vi "balance.vi"() -> ()   [LabVIEW 2013]
uses:
  <vilib>/Analysis/NI_AALBase.lvlib
  <vilib>/Instr/_visa.llb/VISA Configure Serial Port (Instr).vi
  <vilib>/Analysis/3filter.llb/Savitzky-Golay Filter (DBL).vi
  <vilib>/Analysis/3filter.llb/FIR Filter (DBL).vi
  <vilib>/Analysis/3filter.llb/Zero Phase Filter (DBL).vi
  <vilib>/measure/maspectr.llb/FFT Spectrum (Mag-Phase).vi
  <vilib>/measure/NI_MAPro.lvlib
  <vilib>/robotics/Controls/2D Rangefinder/NI_Robotics_2D Rangefinder.xctl
panel:
  in  "PWM":u16(knob) scale=1100.0..1900.0
  in  "Направление\nвращения":dbl=-1.0
  in  "Усиление расчетной фазы":dbl(slide)=0.02993150684931507 scale=0.005..0.04
  in  "Правка фазы":dbl(slide)=105.29268292682927 scale=0.0..360.0
  in  "0 акселер.":dbl
  in  "Выбор т.":bool
  out "max а":i32
  out "по обор.":i32
  out "Рабочий диапозон":waveform(dbl)(graph)
  in  "использование\n ф. сигнала":bool
  out "Расчетные \nзначения":cluster{"angle":dbl[], "distance":dbl[][]}(xcontrol)
  out "Расчетный спектр на основе БПФ":cluster{"f0":dbl, "df":dbl, "magnitude":dbl[]}(graph)
  in  "Сглаживание":T1(ring)
  in  "Правка фазы":dbl(slide) scale=0.0..360.0
  in  "Усиление уровня мигнала":dbl(slide)=0.014857142857142857 scale=0.005..0.02
  out "N об.":i32
  out "Об/мин":dbl(knob) scale=0.0..6000.0
  out "Ф. сигнал\n в полярных \nкоординатах":cluster{"angle":dbl[], "distance":dbl[][]}(xcontrol)
  in  "Вывод\nновых\nданных":bool
  in  "side points":i32(slide)=20 scale=0.0..40.0
  in  "polynomial order":i32(slide)=2 scale=0.0..20.0
  out "Сигнал со стенда":cluster{i32[], dbl[]}[](graph)
  in  "Выбор фильтра":u16(ring) items=["Savetzky-Golay", "Median", "FIR", "Zero Fhase"]
  in  "второй":i32=2
  in  "Установка скорости":u32=115200
  in  "Выбор порта":refnum<visa-resource-name>="COM13"
  out "данные из порта":string
  out "Отфильтрованный сигнал":cluster{i32[], "Filtered X":dbl[]}[](graph)
  in  "stop":bool
  # "0"
  # "180"
  # "F12"
  # "первый"
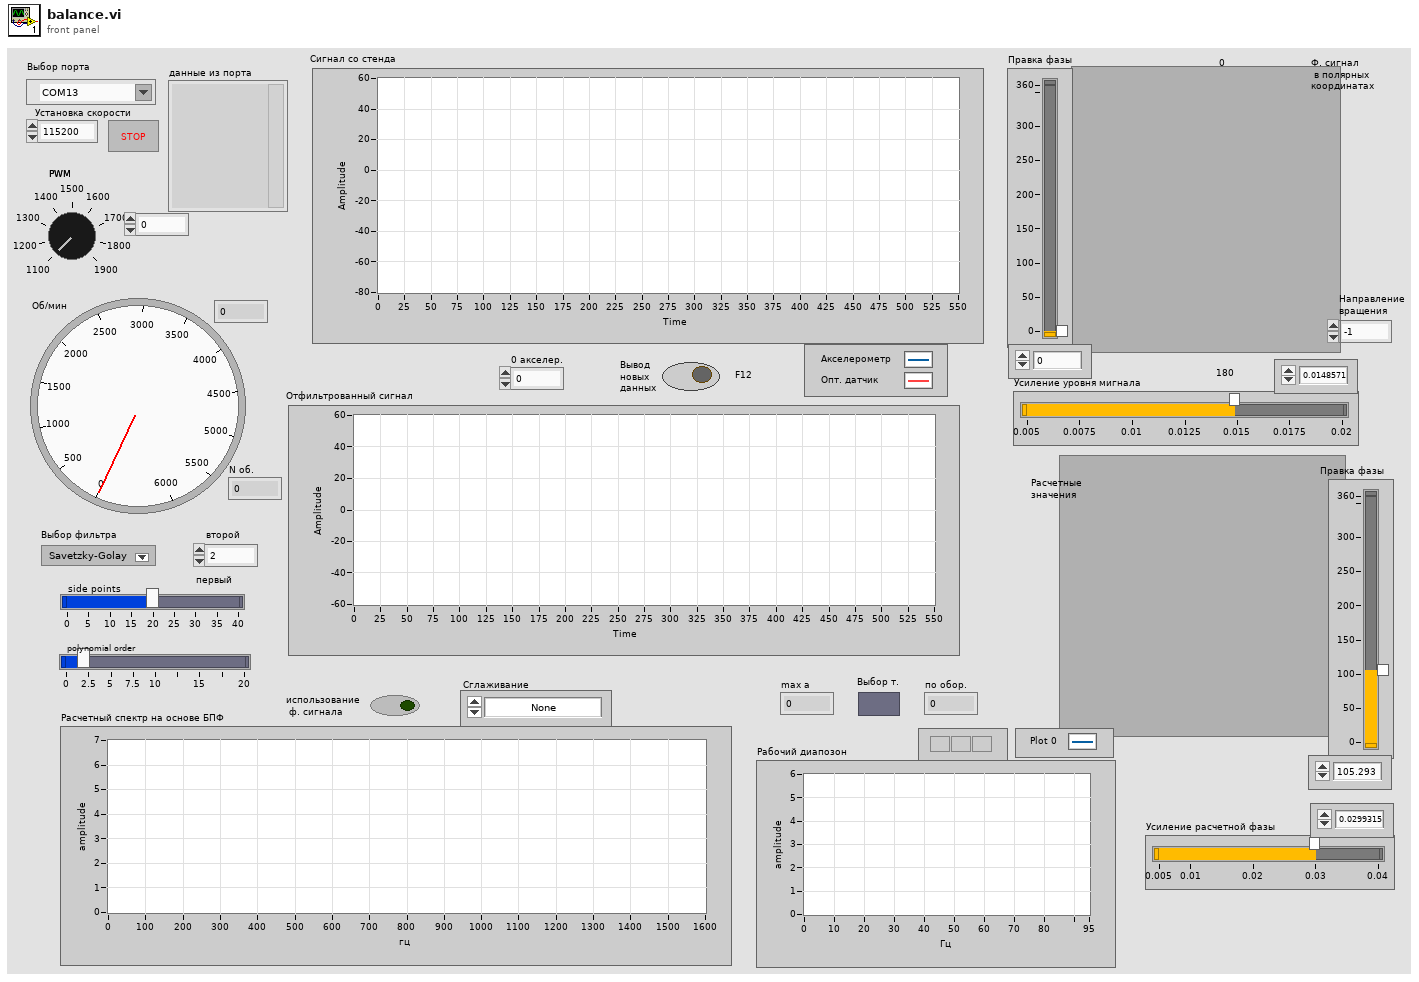
[diagram p1: front panel]
types:
  T1 = enum16{"None ", "Hanning", "Hamming", "Blackman-Harris", "Exact Blackman", "Blackman", "Flat Top", "4 Term B-Harris ", "7 Term B-Harris", "Low Sidelobe"}
  T2 = cluster{"dB On (F)":bool, "unwrap phase (F)":bool, "convert to degree (F)":bool}
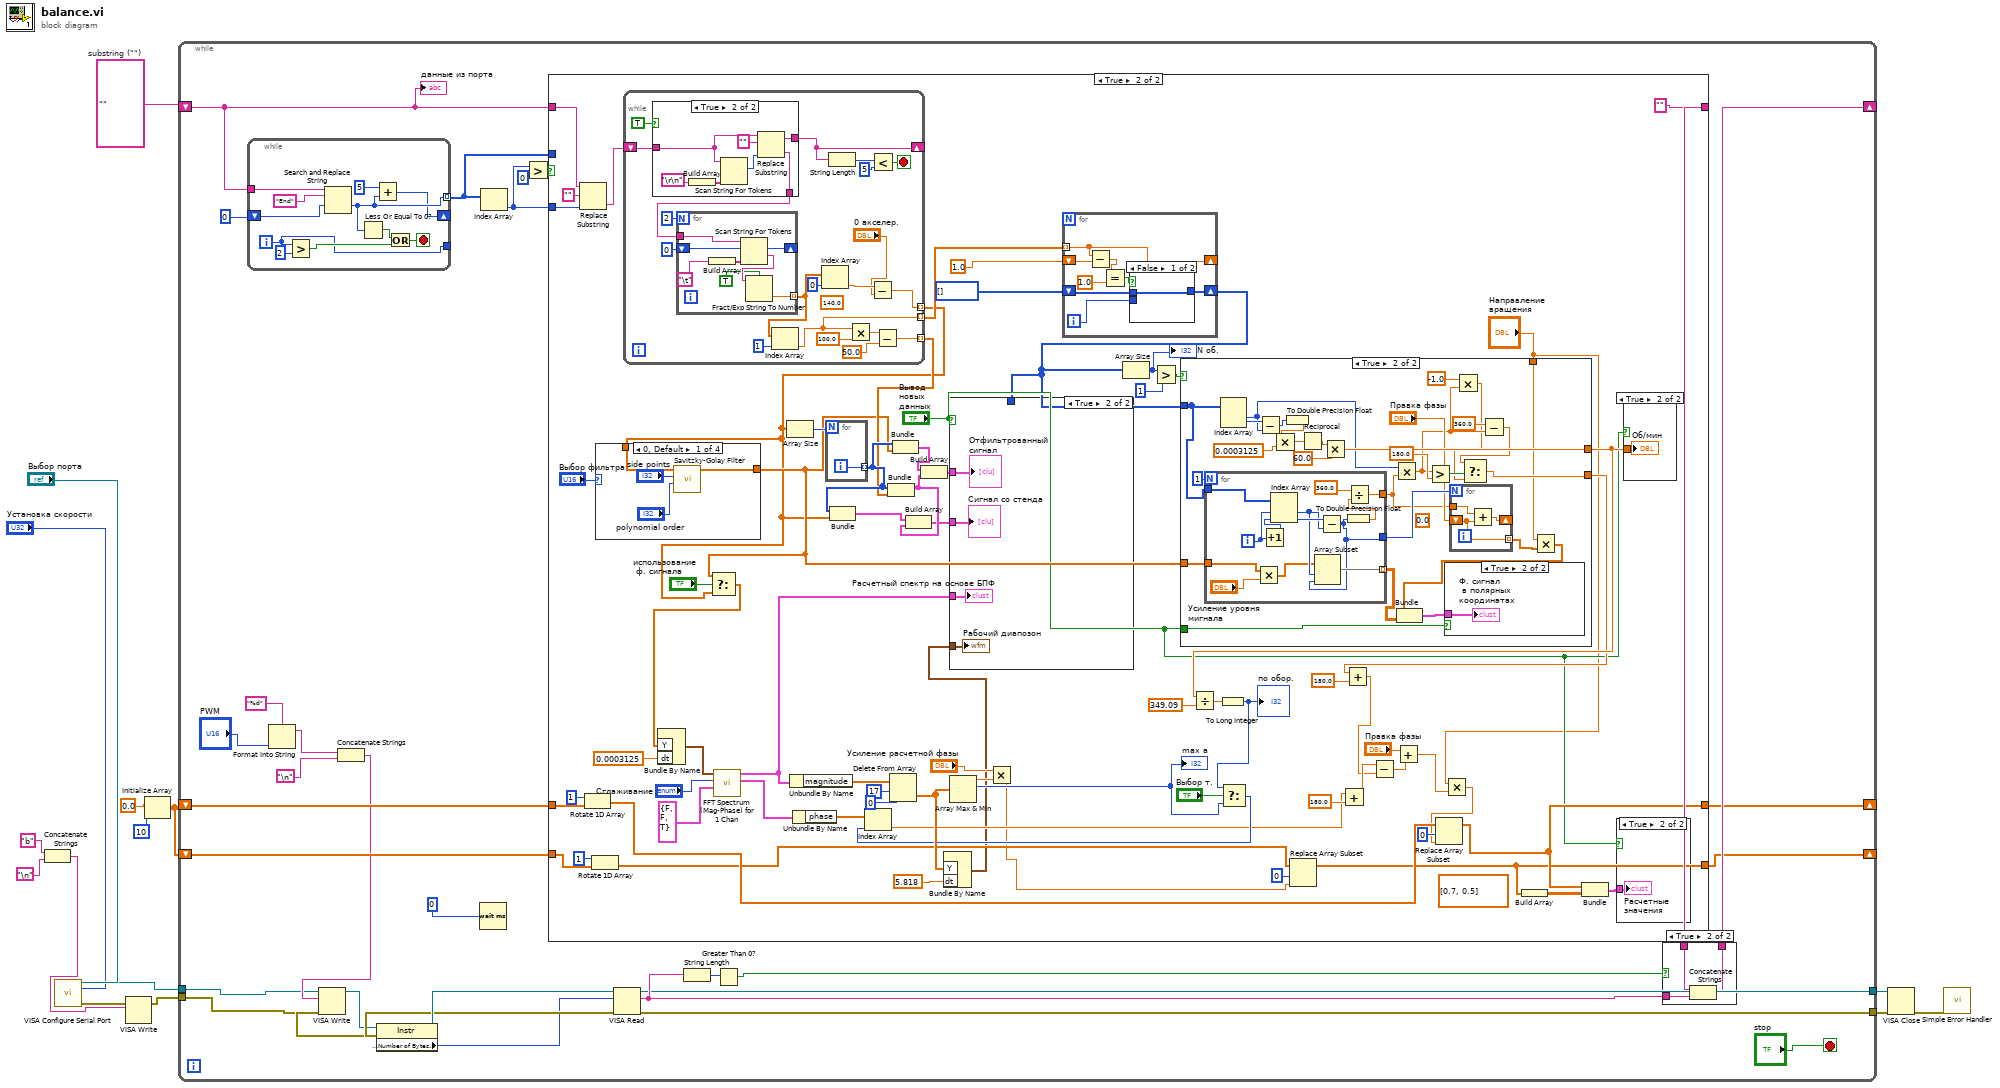
[diagram p0: block diagram]
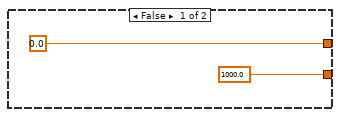
[diagram p6: hidden frame]
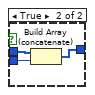
[diagram p8: hidden frame]
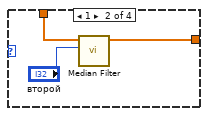
[diagram p10: hidden frame]
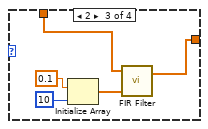
[diagram p11: hidden frame]
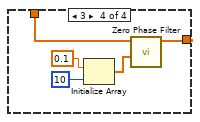
[diagram p12: hidden frame]
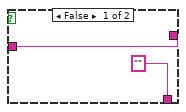
[diagram p13: hidden frame]
diagram:
  w12 = ""  # substring ("")
  n1 = Concatenate Strings("b", "\n") -> (w1:string)
  n2 = call-poly "VISA Configure Serial Port"("VISA resource name"="Выбор порта", "baud rate (9600)"="Установка скорости") -> ("VISA resource name out"=w11:refnum<visa-resource-name>, "error out"=w10:errorcluster)  [unwired: 7 in, 5 out]
  n3 = VISA Write(write buffer=w1) -> ()  [unwired: 2 in, 3 out]
  n4 = Initialize Array(0.0, 10 ("dimension size")) -> (w4:dbl[])
  n5 = while {
    shift-right: [w33] -> _
    shift-left: w12 -> [w30]
    tunnel: w11 -> [w15]
    tunnel: w10 -> [w16]
    tunnel: [w32] -> w8
    tunnel: [w31] -> w7
    shift-right: [w26] -> _
    shift-left: w4 -> [w27]
    shift-right: [w24] -> _
    shift-left: w4 -> [w25]
    stop <- "stop" stop-if-true
    n6 = while {
      tunnel: w30 -> [w256]
      shift-right: [w252] -> _
      shift-left: 0 -> [w251]
      tunnel: [w254] -> w29 mode=indexing
      tunnel: [w246] -> _
      i -> [w246]
      stop <- w247 stop-if-true
      n7 = Greater?(x=w246, y=2) -> (0:w248:bool)
      n8 = Search and Replace String(input string=w256, search string="End", offset=w251) -> (offset past replacement=w254:i32)  [unwired: 5 in, 3 out]
      n9 = Less Or Equal To 0?(x=w254) -> (x <= 0?=w250:bool)
      n10 = Add(x=5, y=w254) -> (x+y=w252:i32)
      n11 = Or(x=w250, y=w248) -> (x .or. y?=w247:bool)
    }
    n12 = Format Into String(format string="%d", "PWM") -> (resulting string=w19:string)  [unwired: 2 in, 1 out]
    n13 = Concatenate Strings(w19, "\n") -> (w17:string)
    n14 = VISA Write(VISA resource name=w15, write buffer=w17, error in (no error)=w16) -> (VISA resource name out=w22:refnum<visa-resource-name>, error out=w23:errorcluster)  [unwired: 1 out]
    n15 = property class="Instr"(reference=w22, error in=w23) -> (reference out=w40:refnum<visa-resource-name>, error out=w39:errorcluster, "Serial Settings:Number of Bytes at Serial Port"=w38:u32)
    n16 = Wait (ms)(milliseconds to wait=u32 0) -> ()  [unwired: 1 out]
    n17 = Index Array(array=w29) -> (element=w28:i32)  [unwired: 1 in]
    n18 = Greater?(x=w28, y=0) -> (0:w41:bool)
    n19 = case shown="True" w41 {
      tunnel: w29 -> [_ _]
      tunnel: [w52 ""] -> w34
      tunnel: w30 -> [w52 w122]
      tunnel: w28 -> [_ w120]
      tunnel: w27 -> [w51 w73]
      tunnel: [w51 w69] -> w26
      tunnel: w25 -> [w50 w67]
      tunnel: [w50 w61] -> w24
      frame False {
      }
      frame True {
        (unwired) dbl[][] [[0.7, 0.5]]
        n20 = Replace Substring(2:w120, 4:"" ("substring (\"\")"), 5:w122) -> (0:w119:string)  [unwired: 1 in, 1 out]
        n21 = Rotate 1D Array(1:w73, 2:1 ("n")) -> (0:w71:dbl[])
        n22 = Rotate 1D Array(1:w67, 2:1 ("n")) -> (0:w65:dbl[])
        n23 = while {
          shift-right: [w223] -> _
          shift-left: w119 -> [w226]
          tunnel: [w211] -> w95 mode=indexing
          tunnel: [w216] -> w103 mode=indexing
          tunnel: [w213] -> w109 mode=indexing
          stop <- w220 stop-if-true
          (unwired) 140.0
          n24 = case shown="True" TRUE {
            tunnel: [w230 w234] -> w223
            tunnel: w226 -> [w230 w233]
            tunnel: ["" w231] -> w225
            frame False {
            }
            frame True {
              n25 = Build Array("\r\n") -> (w236:string[])
              n26 = Scan String For Tokens(6:w236, 9:w233) -> (2:w232:i32)  [unwired: 4 in, 3 out]
              n27 = Replace Substring(2:w232, 4:"" ("substring (\"\")"), 5:w233) -> (0:w231:string, 1:w234:string)  [unwired: 1 in]
            }
          }
          n28 = for {
            N: 2 -> [_]
            tunnel: w225 -> [w244]
            shift-right: [w243] -> _
            shift-left: 0 -> [w242]
            tunnel: [w240] -> w214 mode=indexing
            n29 = Build Array("\t") -> (w245:string[])
            n30 = Scan String For Tokens(6:w245, 8:w242, 9:w244) -> (1:w241:string, 2:w243:i32)  [unwired: 3 in, 2 out]
            n31 = Fract/Exp String To Number(use system decimal point (T)=TRUE, string=w241) -> (number=w240:dbl)  [unwired: 2 in, 1 out]
          }
          n32 = Index Array(array=w214, index=1) -> (element=w213:dbl)
          n33 = Index Array(array=w214, index=0) -> (element=w212:dbl)
          n34 = String Length(string=w223) -> (length=w222:i32)
          n35 = Multiply(x=w213, y=100.0) -> (x*y=w218:dbl)
          n36 = Subtract(x=w212, y="0 акселер.") -> (x-y=w211:dbl)
          n37 = Less?(x=w222, y=5) -> (x < y?=w220:bool)
          n38 = Subtract(x=w218, y=50.0) -> (x-y=w216:dbl)
        }
        n39 = case shown="0, Default" "Выбор фильтра" {
          tunnel: w95 -> [w194 w197 w199 w205]
          tunnel: [w193 w195 w198 w204] -> w96
          frame 0, Default {
            n40 = call-poly <vilib>:"Savitzky-Golay Filter.vi"("polynomial order"="polynomial order", "side points"="side points", "X"=w194) -> ("Filtered X"=w193:dbl[])  [unwired: 7 in, 1 out]
          }
          frame 1 {
            n41 = call <vilib>:"Median Filter.vi"("left rank"="второй", "X"=w197) -> ("Filtered X"=w195:dbl[])  [unwired: 8 in, 1 out]
          }
          frame 2 {
            n42 = Initialize Array(0.1 ("element"), 10 ("dimension size")) -> (w200:dbl[])
            n43 = call-poly <vilib>:"FIR Filter.vi"("FIR Coefficients"=w200, "X"=w199) -> ("Filtered X"=w198:dbl[])  [unwired: 2 in, 1 out]
          }
          frame 3 {
            n44 = Initialize Array(0.1 ("element"), 10 ("dimension size")) -> (w206:dbl[])
            n45 = call-poly <vilib>:"Zero Phase Filter.vi"("Forward Coefficients"=w206, "X"=w205) -> ("Filtered X"=w204:dbl[])  [unwired: 8 in, 1 out]
          }
        }
        n46 = Select(t=w96, s="использование\n ф. сигнала", f=w95) -> (s? t:f=w94:dbl[])
        n47 = Bundle By Name("Y"=w94, "dt"=0.0003125) -> (w98:waveform(dbl))  [unwired: 1 in]
        n48 = call-poly <vilib>:"FFT Spectrum (Mag-Phase) for 1 Chan.vi"("view"=T2 {"dB On (F)"=FALSE, "unwrap phase (F)"=FALSE, "convert to degree (F)"=TRUE}, "window"="Сглаживание", "time signal"=w98) -> ("phase"=w83:cluster{"f0":dbl, "df":dbl, "phase":dbl[]}, "magnitude"=w59:cluster{"f0":dbl, "df":dbl, "magnitude":dbl[]})  [unwired: 4 in, 3 out]
        n49 = Array Size(array=w95) -> (size(s)=w107:i32)
        n50 = Unbundle By Name(w59) -> ("magnitude"=w93:dbl[])
        n51 = Unbundle By Name(w83) -> ("phase"=w97:dbl[])
        n52 = for {
          N: w107 -> [_]
          tunnel: [w208] -> w117 mode=indexing
          i -> [w208]
        }
        n53 = Bundle(w117, w95) -> (w118:cluster{i32[], dbl[]})  [unwired: 1 in]
        n54 = Bundle(w117, w103) -> (w116:cluster{i32[], dbl[]})  [unwired: 1 in]
        n55 = Delete From Array(array=w93, length=17, index=0) -> (deleted portion=w88:dbl[])  [unwired: 1 out]
        n56 = Bundle(w117, "Filtered X"=w96) -> (w124:cluster{i32[], "Filtered X":dbl[]})  [unwired: 1 in]
        n57 = Build Array(w118, w116) -> (w115:cluster{i32[], dbl[]}[])
        n58 = Build Array(w124, w116) -> (w106:cluster{i32[], "Filtered X":dbl[]}[])
        n59 = Bundle By Name("Y"=w88, "dt"=5.818) -> (w57:waveform(dbl))  [unwired: 1 in]
        n60 = Array Max & Min(array=w88) -> (max value=w64:dbl, max index (indices)=w85:i32)  [unwired: 2 out]
        "max а" <- w85
        n61 = Multiply(x="Усиление расчетной фазы", y=w64) -> (x*y=w62:dbl)
        n62 = for {
          tunnel: w109 -> [w181] mode=indexing
          shift-right: [w181] -> _
          shift-left: 1.0 -> [w182]
          shift-right: [w175] -> w56
          shift-left: i32[] [] -> [w176]
          i -> [w177]
          n63 = Subtract(x=w181, y=w182) -> (x-y=w180:dbl)
          n64 = Equal?(x=w180, y=1.0) -> (x = y?=w178:bool)
          n65 = case shown="False" w178 {
            tunnel: w177 -> [_ w186]
            tunnel: w176 -> [w183 w185]
            tunnel: [w183 w184] -> w175
            frame False {
            }
            frame True {
              n66 = Build Array (concatenate)(w185, w186) -> (w184:i32[])
            }
          }
        }
        n67 = case shown="True" "Вывод\nновых\nданных" {
          tunnel: w106 -> [_ w190]
          tunnel: w115 -> [_ w189]
          tunnel: w59 -> [_ w188]
          tunnel: w57 -> [_ w187]
          tunnel: w56 -> [_ _]
          frame False {
          }
          frame True {
            "Отфильтрованный сигнал" <- w190
            "Сигнал со стенда" <- w189
            "Расчетный спектр на основе БПФ" <- w188
            "Рабочий диапозон" <- w187
          }
        }
        n68 = Array Size(array=w56) -> (size(s)=w108:i32)
        "N об." <- w108
        n69 = Greater?(x=w108, y=1) -> (0:w110:bool)
        n70 = case shown="True" w110 {
          tunnel: w56 -> [_ w151]
          tunnel: [0.0 w152] -> w102
          tunnel: w96 -> [_ w142]
          tunnel: "Вывод\nновых\nданных" -> [_ w144]
          tunnel: [1000.0 w132] -> w82
          tunnel: "Направление\nвращения" -> [_ w129]
          frame False {
          }
          frame True {
            (unwired) 0.0
            n71 = for {
              N: 1 -> [_]
              tunnel: w151 -> [w172]
              tunnel: w142 -> [w164]
              tunnel: [w167] -> w146 mode=indexing
              tunnel: [w166] -> w145
              tunnel: [w165] -> w141
              i -> [w173]
              n72 = Multiply(x=w164, y="Усиление уровня мигнала") -> (x*y=w163:dbl[])
              n73 = Increment(x=w173) -> (x+1=w174:i32)
              n74 = Index Array(array=w172, index #1=w173, index #2=w174) -> (element #1=w168:i32, element #2=w169:i32)
              n75 = Subtract(x=w169, y=w168) -> (x-y=w166:i32)
              n76 = Array Subset(array=w163, index=w168, length=w166) -> (w167:dbl[])
              n77 = To Double Precision Float(number=w166) -> (double precision float=w170:dbl)
              n78 = Divide(x=360.0, y=w170) -> (x/y=w165:dbl)
            }
            n79 = Index Array(array=w151) -> (element #1=w140:i32, element #2=w157:i32)  [unwired: 2 in]
            n80 = Subtract(x=w157, y=w140) -> (x-y=w150:i32)
            n81 = To Double Precision Float(number=w150) -> (double precision float=w149:dbl)
            n82 = Multiply(x=w149, y=0.0003125 ("dt")) -> (x*y=w155:dbl)
            n83 = Reciprocal(x=w155) -> (1/x=w154:dbl)
            n84 = Multiply(x=w154, y=60.0) -> (x*y=w152:dbl)
            n85 = Multiply(x=w140, y=w141) -> (x*y=w135:dbl)
            n86 = Greater?(x=w135, y=180.0) -> (0:w138:bool)
            n87 = for {
              N: w145 -> [_]
              shift-right: [w160] -> _
              shift-left: "Правка фазы" -> [w159]
              tunnel: w141 -> [w161]
              tunnel: [w159] -> w131 mode=indexing
              n88 = Add(x=w161, y=w159) -> (x+y=w160:dbl)
            }
            n89 = Multiply(x=-1.0, y=w135) -> (x*y=w133:dbl)
            n90 = Subtract(x=360.0, y=w135) -> (x-y=w136:dbl)
            n91 = Select(t=w136, s=w138, f=w133) -> (s? t:f=w132:dbl)
            n92 = Multiply(x=w129, y=w131) -> (x*y=w130:dbl[])
            n93 = Bundle(w130, w146) -> (w147:cluster{dbl[], dbl[][]})  [unwired: 1 in]
            n94 = case shown="True" w144 {
              tunnel: w147 -> [_ w158]
              frame False {
              }
              frame True {
                "Ф. сигнал\n в полярных \nкоординатах" <- w158
              }
            }
          }
        }
        n95 = Divide(x=w102, y=349.09) -> (x/y=w100:dbl)
        n96 = To Long Integer(number=w100) -> (32bit integer=w86:i32)
        "по обор." <- w86
        n97 = Select(t=w86, s="Выбор т.", f=w85) -> (s? t:f=w84:i32)
        n98 = Index Array(array=w97, index=w84) -> (element=w79:dbl)
        n99 = Replace Array Subset(array=w65, new element=w62, index=0) -> (w61:dbl[])
        n100 = Add(x=w79, y=180.0) -> (x+y=w78:dbl)
        n101 = Add(x=w82, y=180.0) -> (x+y=w77:dbl)
        n102 = Subtract(x=w78, y=w77) -> (x-y=w75:dbl)
        n103 = Add(x="Правка фазы", y=w75) -> (x+y=w53:dbl)
        n104 = Multiply(x="Направление\nвращения", y=w53) -> (x*y=w55:dbl)
        n105 = Replace Array Subset(array=w71, new element=w55, index=0) -> (w69:dbl[])
        n106 = Build Array(w61) -> (w60:dbl[][])
        n107 = Bundle(w69, w60) -> (w99:cluster{dbl[], dbl[][]})  [unwired: 1 in]
        n108 = case shown="True" "Вывод\nновых\nданных" {
          tunnel: w99 -> [_ w125]
          frame False {
          }
          frame True {
            "Расчетные \nзначения" <- w125
          }
        }
        n109 = case shown="True" "Вывод\nновых\nданных" {
          tunnel: w102 -> [_ w126]
          frame False {
          }
          frame True {
            "Об/мин" <- w126
          }
        }
      }
    }
    n110 = VISA Read(VISA resource name=w40, byte count=w38, error in (no error)=w39) -> (VISA resource name out=w32:refnum<visa-resource-name>, read buffer=w35:string, error out=w31:errorcluster)  [unwired: 1 out]
    n111 = String Length(string=w35) -> (length=w37:i32)
    n112 = Greater Than 0?(x=w37) -> (x > 0?=w36:bool)
    n113 = case shown="True" w36 {
      tunnel: w35 -> [_ w47]
      tunnel: w34 -> [w46 w49]
      tunnel: [w46 w48] -> w33
      frame False {
      }
      frame True {
        n114 = Concatenate Strings(w49, w47) -> (w48:string)
      }
    }
    "данные из порта" <- w30
  }
  n115 = VISA Close(VISA resource name=w8, error in (no error)=w7) -> (error out=w9:errorcluster)
  n116 = call <vilib>:"Simple Error Handler.vi"("error in (no error)"=w9) -> ()  [unwired: 1 in, 8 out]
